vi "Initialize Camera Servos.vi"   [LabVIEW 2020]
uses:
  <vilib>/Rock Robotics/SystemInterfaces/DIO/FPGA_DIOPWMChannel.ctl
types:
  T1 = typedef "FPGA_DIOPWMChannel.ctl" = enum8{"PWM 0", "PWM 1", "PWM 2", "PWM 3", "PWM 4", "PWM 5", "PWM 6", "PWM 7", "PWM 8", "PWM 9", "PWM MXP 0", "PWM MXP 1", "PWM MXP 2", "PWM MXP 3", "PWM MXP 4", "PWM MXP 5", "PWM MXP 6", "PWM MXP 7", "PWM MXP 8", "PWM MXP 9", "Invalid"}
  T2 = typedef "WPI_ServoDeviceRef.ctl" = cluster{"DeviceStatus":errorcluster, "PWM Channel":T1, "DeadBand":T3}
  T3 = typedef "WPI_PWMDeadband.ctl" = cluster{"Name":string, "maxPositivePwm":i32, "minPositivePwm":i32, "centerPwm":i32, "maxNegativePwm":i32, "minNegativePwm":i32, "angularRange":u16}
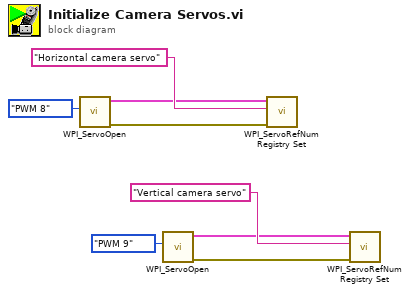
[diagram p0: block diagram]
diagram:
  n1 = call <vilib>:"WPI_ServoOpen.vi"("PWM Channel"=FPGA_DIOPWMChannel."PWM 8") -> ("error out"=w2:errorcluster, "ServoDeviceRef"=w3:T2)  [unwired: 9 in]
  n2 = call <vilib>:"WPI_ServoOpen.vi"("PWM Channel"=FPGA_DIOPWMChannel."PWM 9") -> ("error out"=w6:errorcluster, "ServoDeviceRef"=w7:T2)  [unwired: 9 in]
  n3 = call <vilib>:"WPI_ServoRefNum Registry Set.vi"("error in (no error)"=w2, "refnum name"="Horizontal camera servo", "ServoDeviceRef"=w3) -> ()  [unwired: 7 in, 2 out]
  n4 = call <vilib>:"WPI_ServoRefNum Registry Set.vi"("error in (no error)"=w6, "refnum name"="Vertical camera servo", "ServoDeviceRef"=w7) -> ()  [unwired: 7 in, 2 out]
